vi "Add XY (multiple).vi"(8 "error in (no error)":errorcluster, 9 "y":cluster{"X-array":dbl[], "Y-array":dbl[]}, 10 "x":cluster{"X-array":dbl[], "Y-array":dbl[]}, 11 "XY-data":cluster{"X-array":dbl[], "Y-array":dbl[]}[](array[cluster]) {"Y-array" format="%.2p"; "X-array" format="%.2p"}) -> (0 "error out":errorcluster, 3 "XY-data out":cluster{"X-array":dbl[], "Y-array":dbl[]}[](array[cluster]) {"Y-array" format="%.2p"; "X-array" format="%.2p"})   [LabVIEW 2019, in "xy_utilities.lvlib"]
doc: "Add <b>x</b>'s x array to the x array of <b>XY-data</b>\nAdd <b>y</b>'s y array to the y array of <b>XY-data</b>\n\nWire data to the data input to determine the polymorphic instance to use or manually select the instance."
uses:
  xy_utilities.lvlib
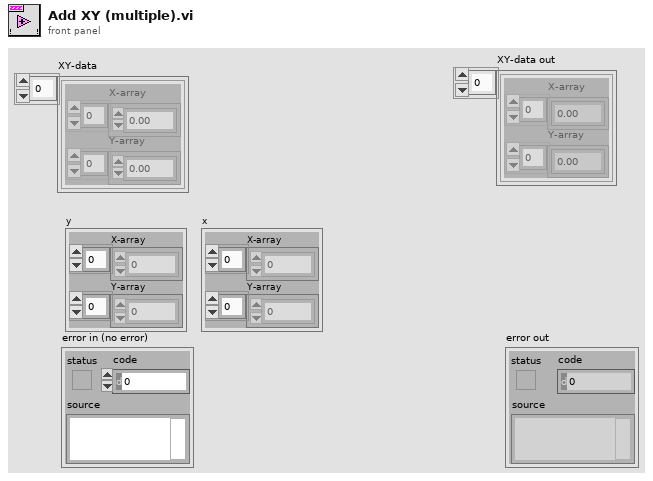
[diagram p1: front panel]
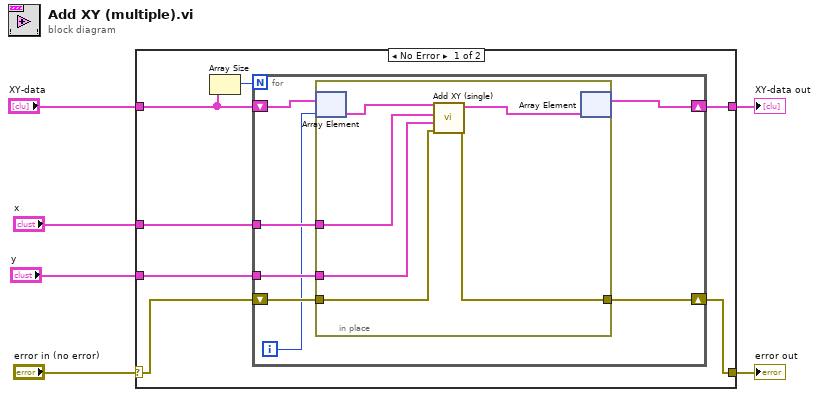
[diagram p0: block diagram]
diagram:
  n1 = case shown="No Error" "error in (no error)" {
    selector: "error in (no error)" -> [w10 w27]
    tunnel: [w9 w27] -> w1
    tunnel: "XY-data" -> [w7 w28]
    tunnel: [w13 w28] -> w4
    tunnel: "y" -> [w12 _]
    tunnel: "x" -> [w11 _]
    frame No Error {
      n2 = Array Size(array=w7) -> (size(s)=w8:i32)
      n3 = for {
        N: w8 -> [_]
        tunnel: w12 -> [w20]
        tunnel: w11 -> [w17]
        shift-right: [w18] -> w9
        shift-left: w10 -> [w19]
        shift-right: [w14] -> w13
        shift-left: w7 -> [w16]
        i -> [w15]
        n4 = in-place {
          in-place-border: w20 -> [w26]
          in-place-border: w19 -> [w25]
          in-place-border: [w24] -> w18
          in-place-border: w17 -> [w23]
          n5 = in-place-array #1(w16, w15) -> (w22:cluster{"X-array":dbl[], "Y-array":dbl[]})
          n6 = call "Add XY (single).vi"("error in (no error)"=w25, "y"=w26, "x"=w23, "XY-data"=w22) -> ("error out"=w24:errorcluster, "XY-data out"=w21:cluster{"X-array":dbl[], "Y-array":dbl[]})  [unwired: 6 in]
          n7 = in-place-array #1(w21) -> (w14:cluster{"X-array":dbl[], "Y-array":dbl[]}[])  [unwired: 1 out]
        }
      }
    }
    frame Error {
    }
  }
  "error out" <- w1
  "XY-data out" <- w4
